vi "ProgressPopup.vi"(10 "Message":string) -> ()   [LabVIEW 2020, in "hse-ui.lvlib"]
doc: "____\nHAMPEL SOFTWARE ENGINEERING v3.8.0 (2023-12-18 14:41)"
uses:
  hse-ui.lvlib
  FPControl/FPControl_Actions.ctl
panel:
  in  "Stop":bool
  out "Message out":string
  out "Progress":i32(slide) scale=0.0..100.0
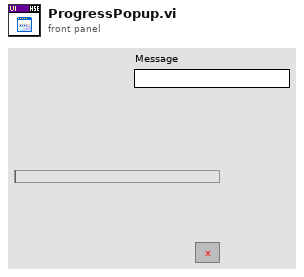
[diagram p1: front panel]
types:
  T1 = typedef "hse-ui.lvlib/FPControl_Actions.ctl" = enum16{"Open", "Hide", "Close", "Bring To Front", "Center", "Minimize", "Maximize"}
  T2 = typedef "LVRectTypeDef.ctl" = cluster{"Left":i16, "Top":i16, "Right":i16, "Bottom":i16}
  T3 = cluster{"left":i16, "top":i16, "right":i16, "bottom":i16}
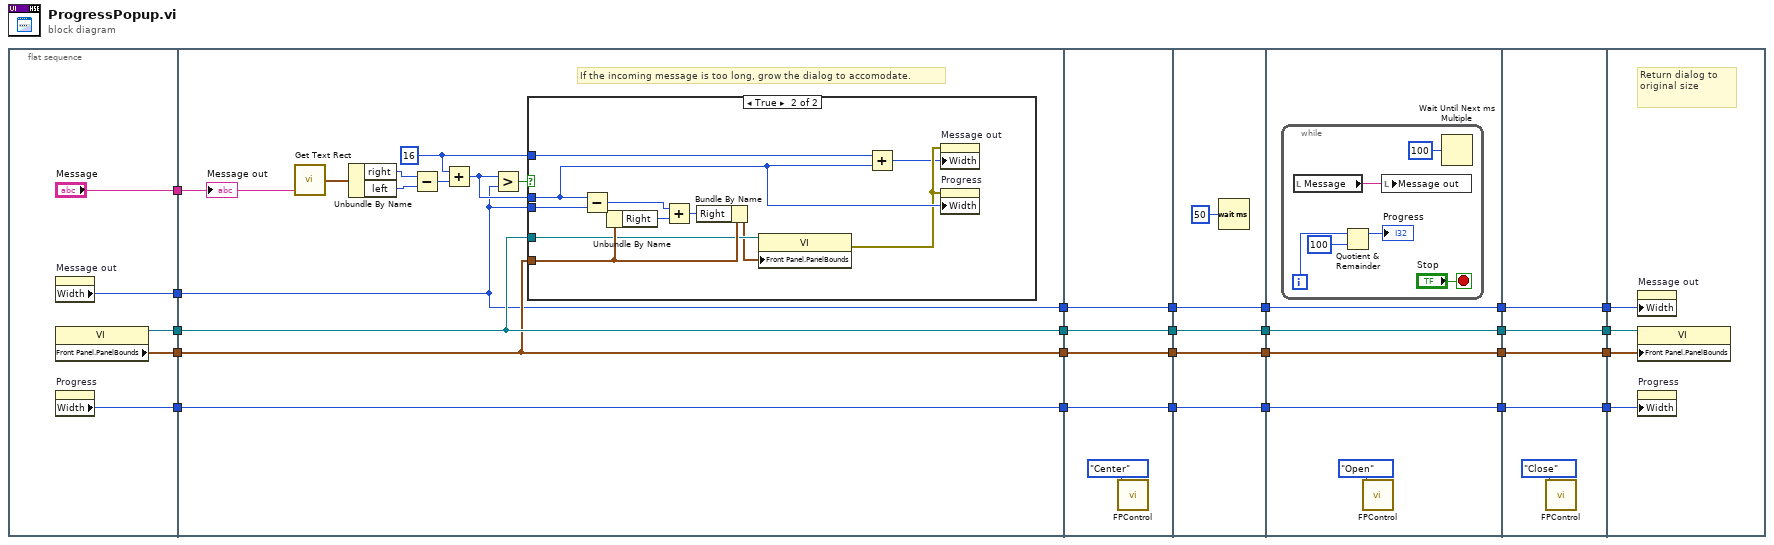
[diagram p0: block diagram]
diagram:
  n1 = flat-sequence {
    tunnel: ["Message"] -> w5
    tunnel: [w29] -> w4
    tunnel: [w28] -> w3
    tunnel: [w27] -> w2
    tunnel: [w26] -> w1
    tunnel: [w33] -> w23
    tunnel: [w35] -> w20
    tunnel: [w34] -> w17
    tunnel: [w32] -> w14
    tunnel: w5 -> [w31]
    tunnel: w4 -> [w35]
    tunnel: w3 -> [w34]
    tunnel: w2 -> [w33]
    tunnel: w1 -> [w32]
    tunnel: [w58] -> w13
    tunnel: w23 -> [w58]
    tunnel: [w57] -> w11
    tunnel: w20 -> [w57]
    tunnel: [w56] -> w9
    tunnel: w17 -> [w56]
    tunnel: [w55] -> w7
    tunnel: w14 -> [w55]
    tunnel: w13 -> [w63]
    tunnel: [w63] -> w12
    tunnel: w11 -> [w62]
    tunnel: [w62] -> w10
    tunnel: w9 -> [w61]
    tunnel: [w61] -> w8
    tunnel: w7 -> [w60]
    tunnel: [w60] -> w6
    tunnel: [w68] -> w24
    tunnel: w12 -> [w68]
    tunnel: [w67] -> w21
    tunnel: w10 -> [w67]
    tunnel: [w66] -> w18
    tunnel: w8 -> [w66]
    tunnel: [w65] -> w15
    tunnel: w6 -> [w65]
    tunnel: [w79] -> w25
    tunnel: w24 -> [w79]
    tunnel: [w78] -> w22
    tunnel: w21 -> [w78]
    tunnel: [w77] -> w19
    tunnel: w18 -> [w77]
    tunnel: [w76] -> w16
    tunnel: w15 -> [w76]
    tunnel: w25 -> [w83]
    tunnel: w22 -> [w82]
    tunnel: w19 -> [w81]
    tunnel: w16 -> [w80]
    frame #0 {
      n2 = property on="Message out" class="Str"() -> ("Width"=w27:u32)  [unwired: 2 in, 2 out]
      n3 = property class="VI"() -> (reference out=w29:refnum<vi>, "Front Panel.PanelBounds"=w28:T2)  [unwired: 2 in, 1 out]
      n4 = property on="Progress" class="Slide (strict)"() -> ("Width"=w26:u32)  [unwired: 2 in, 2 out]
    }
    frame #1 {
      w36 = i16 16 ("y")
      # "If the incoming message is too long, grow the dialog to accomodate."
      n5 = call <vilib>:"Get Text Rect.vi"("text"=w31) -> ("rect"=w42:T3)  [unwired: 8 in]
      n6 = Unbundle By Name(w42) -> ("right"=w41:i16, "left"=w40:i16)
      n7 = Subtract(x=w41, y=w40) -> (x-y=w37:i16)
      n8 = Add(x=w36, y=w37) -> (x+y=w39:i16)
      n9 = Greater?(x=w39, y=w33) -> (0:w38:bool)
      n10 = case shown="True" w38 {
        tunnel: w39 -> [_ w53]
        tunnel: w34 -> [_ w52]
        tunnel: w35 -> [_ w51]
        tunnel: w33 -> [_ w50]
        tunnel: w36 -> [_ w43]
        frame False {
        }
        frame True {
          n11 = Subtract(x=w53, y=w50) -> (x-y=w45:u32)
          n12 = Unbundle By Name(w52) -> ("Right"=w46:i16)
          n13 = Add(x=w45, y=w46) -> (x+y=w49:u32)
          n14 = Bundle By Name(cluster=w52, "Right"=w49) -> (w48:T2)
          n15 = property class="VI"(reference=w51, "Front Panel.PanelBounds"=w48) -> (error out=w47:errorcluster)  [unwired: 1 in, 1 out]
          n16 = Add(x=w43, y=w53) -> (x+y=w44:i16)
          n17 = property on="Message out" class="Str"(error in=w47, "Width"=w44) -> ()  [unwired: 1 in, 2 out]
          n18 = property on="Progress" class="Slide (strict)"(error in=w47, "Width"=w53) -> ()  [unwired: 1 in, 2 out]
        }
      }
      "Message out" <- w31
    }
    frame #2 {
      n19 = call "FPControl.vi"("Function"=FPControl_Actions."Center") -> ()  [unwired: 1 in, 10 out]
    }
    frame #3 {
      n20 = Wait (ms)(milliseconds to wait=u32 50) -> ()  [unwired: 1 out]
    }
    frame #4 {
      n21 = while {
        i -> [w74]
        stop <- "Stop" stop-if-true
        n22 = local read "Message"() -> (w69:string)
        n23 = Quotient & Remainder(x=w74, y=100) -> (x-y*floor(x/y)=→"Progress":i32)  [unwired: 1 out]
        n24 = local write "Message out"(w69) -> ()
        n25 = Wait Until Next ms Multiple(millisecond multiple=u32 100) -> ()  [unwired: 1 out]
      }
      n26 = call "FPControl.vi"("Function"=FPControl_Actions."Open") -> ()  [unwired: 1 in, 10 out]
    }
    frame #5 {
      n27 = call "FPControl.vi"("Function"=FPControl_Actions."Close") -> ()  [unwired: 1 in, 10 out]
    }
    frame #6 {
      # "Return dialog to original size"
      n28 = property on="Message out" class="Str"("Width"=w83) -> ()  [unwired: 2 in, 2 out]
      n29 = property class="VI"(reference=w82, "Front Panel.PanelBounds"=w81) -> ()  [unwired: 1 in, 2 out]
      n30 = property on="Progress" class="Slide (strict)"("Width"=w80) -> ()  [unwired: 2 in, 2 out]
    }
  }
